vi "AT Command A.vi"(8 "error in (no error)":errorcluster, 10 "Feature":string, 11 "Handle":i32) -> (0 "error out":errorcluster, 3 "Status":i32)   [LabVIEW 2019]
doc: "Command\n\nOutput:\n I32 Status\n\nInput:\n I32 Handle\n String Feature \n\nThis function will trigger the specified command feature to execute. An error will be returned if the feature is currently not writable, not a command feature or is not implemented by the camera."
uses:
  atcoreA.dll
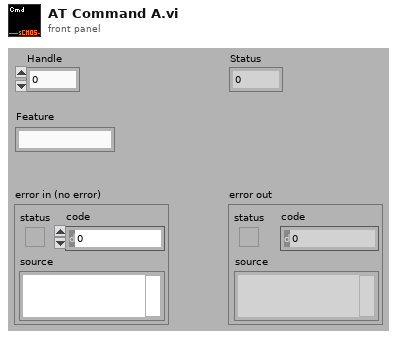
[diagram p1: front panel]
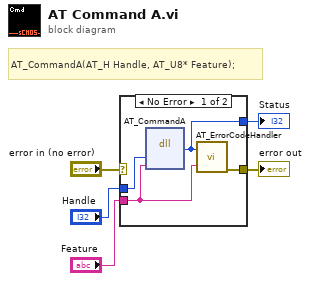
[diagram p0: block diagram]
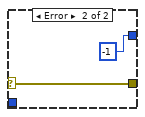
[diagram p2: hidden frame]
diagram:
  # "AT_CommandA(AT_H Handle, AT_U8* Feature);"
  n1 = case shown="No Error" "error in (no error)" {
    selector: "error in (no error)" -> [_ w11]
    tunnel: [w8 w11] -> w5
    tunnel: "Handle" -> [w9 _]
    tunnel: "Feature" -> [w6 _]
    tunnel: [w7 -1] -> w1
    frame No Error {
      n2 = dll-call lib="atcoreA.dll" fn="AT_CommandA"("Handle"=w9, "Feature"=w6) -> ("Status"=w7:i32)  [unwired: 5 in, 2 out]
      n3 = call <userlib>:"AT_ErrorCodeHandler.vi"("Error"=w7, "Feature Name"=w6) -> ("error out"=w8:errorcluster)  [unwired: 5 in]
    }
    frame Error {
    }
  }
  "Status" <- w1
  "error out" <- w5
